vi "subGetReferenceRefs.vi"(8 "error in (no error)":errorcluster, 11 "Refnum in":refnum<k20>) -> (0 "error out":errorcluster, 2 "node result array":refnum<k20>[](array[refnum]), 3 "Refnum out":refnum<k20>)   [LabVIEW 2020, in "DefaultExtensions.lvlib" / "CDefaultRuleFileParser.lvclass"]
uses:
  CDefaultRuleFileParser.lvclass
  <vilib>/xml/NI_XML.lvlib
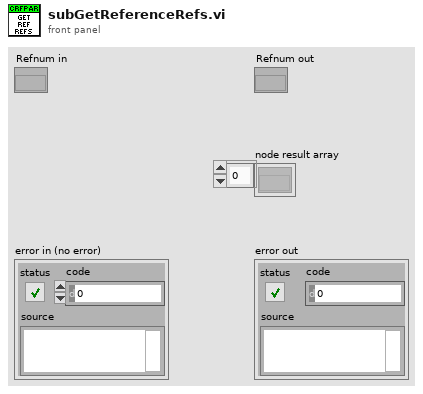
[diagram p1: front panel]
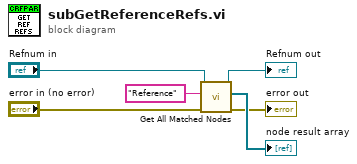
[diagram p0: block diagram]
diagram:
  n1 = call <vilib>:"Get All Matched Nodes.vi"("error in (no error)"="error in (no error)", "XPath expression"="Reference", "node in"="Refnum in") -> ("error out"=→"error out":errorcluster, "node result array"=→"node result array":refnum<k20>[], "node out"=→"Refnum out":refnum<k20>)  [unwired: 6 in]
